vi "main-pressure-logger.vi"() -> ()   [LabVIEW 2016]
uses:
  <vilib>/addons/h5labview2/base/hid_t.ctl
  <vilib>/NI/Modbus Library/API/Wrapper/Create Serial Master.vi
  <vilib>/NI/Modbus Library/API/Master/Modbus Master.lvclass
  <vilib>/NI/Modbus Library/API/Wrapper/API Main.lvlib
  <vilib>/addons/h5labview2/dataset/H5D.lvlib
  <vilib>/addons/h5labview2/file/H5F.lvlib
panel:
  in  "log folder":path=path "C:/Users/LocalAdmin/Documents/omicron-rack/pressure-logs"
  out "Waveform Chart":waveform(sgl)[](graph)
  out "lt":sgl format="%_3e"
  in  "quit":bool
  out "prevacuum":sgl format="%#.3g"
  out "prep":sgl caption="PREP" format="%_3e"
  # "mbar"
  # "mbar"
  # "prep"
  # "lt"
  # "(mbar)"
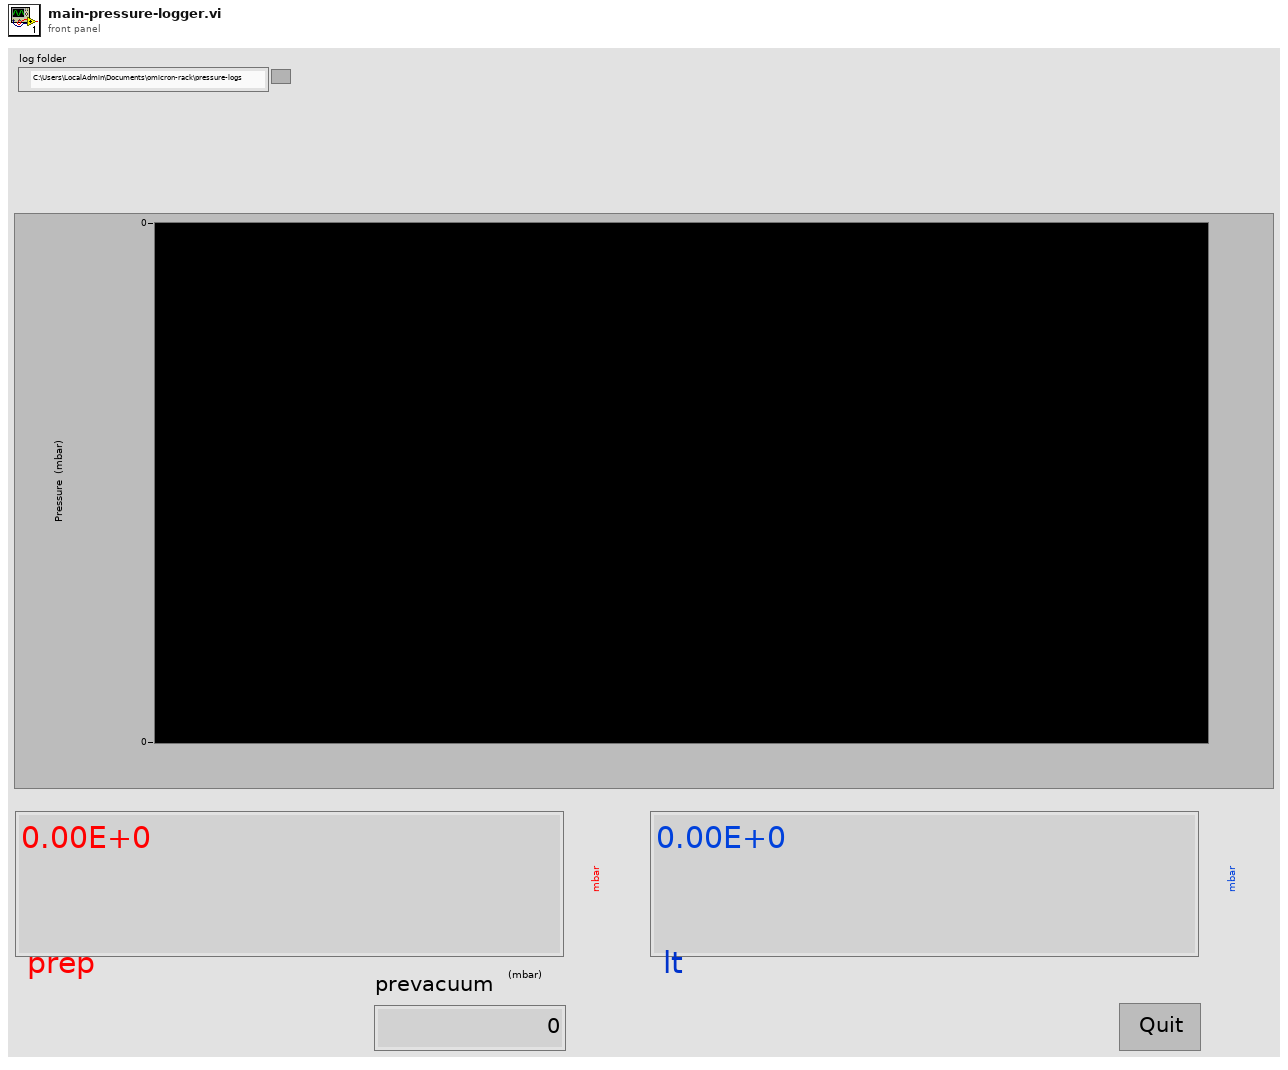
[diagram p1: front panel]
types:
  T1 = typedef "hid_t.ctl" = i32
  T2 = enum16{"open", "replace", "create", "open or create", "replace or create", "replace or create with confirmation"}
  T3 = cluster{"timestamp":i64, "time <19>":string, "prep":sgl, "lt":sgl, "prevacuum":sgl}
  T4 = cluster{"timestamp":i64, "time <19>":string, "prep":sgl, "lt":sgl, "prevacuum":sgl}[]
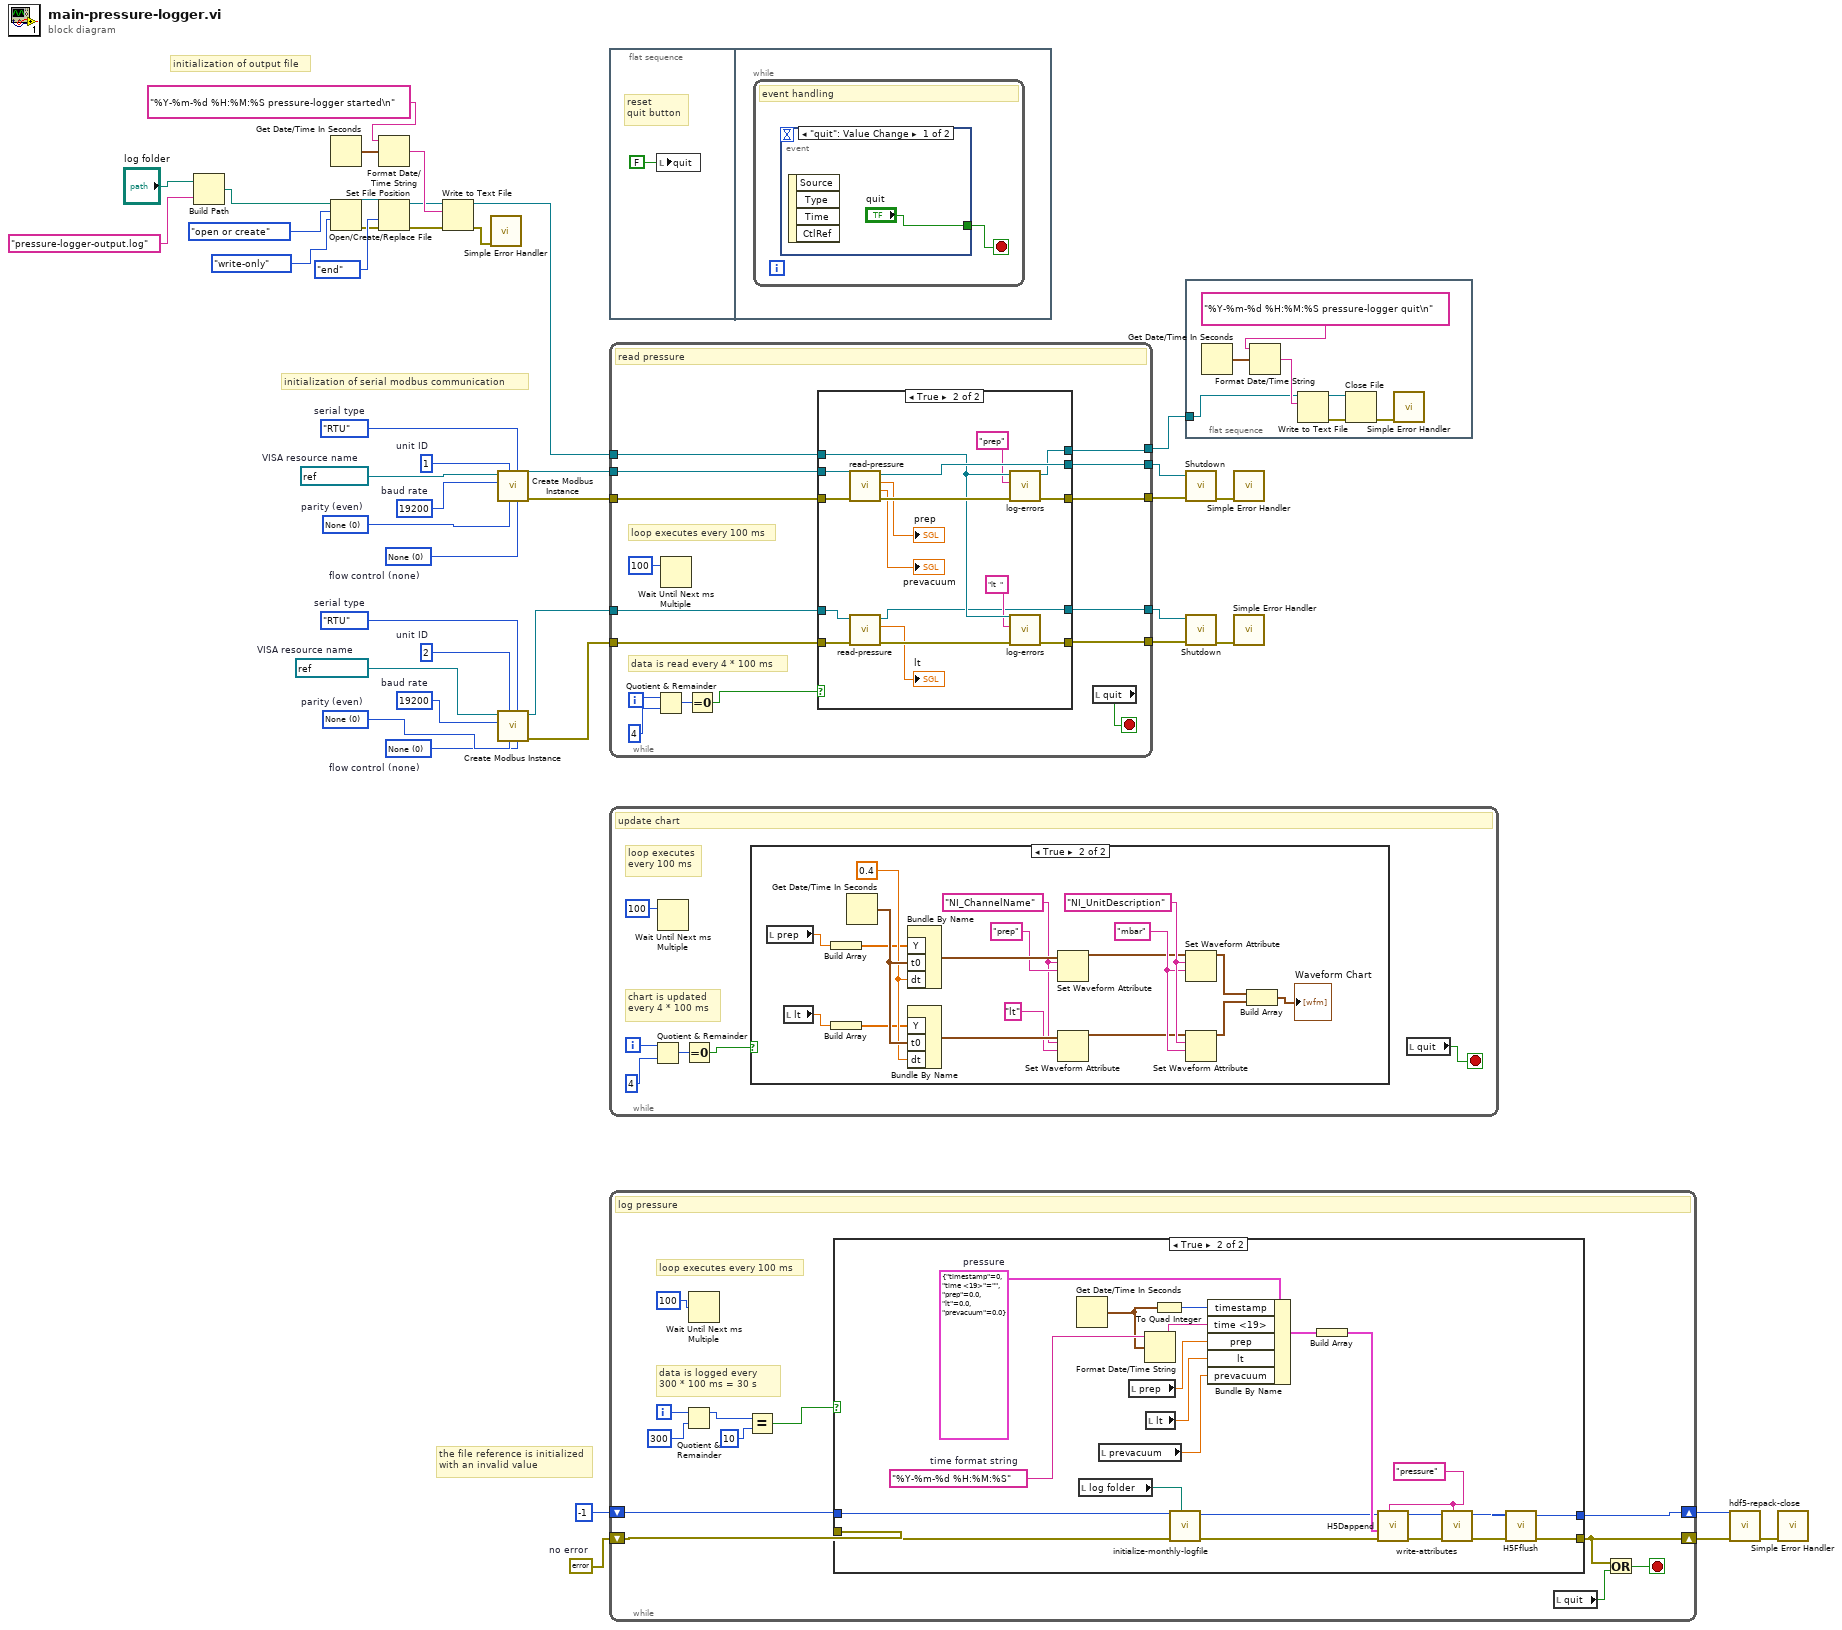
[diagram p0: block diagram]
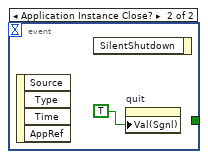
[diagram p3: hidden frame]
diagram:
  w1 = errorcluster {"status"=FALSE, "code"=0, "source"=""}  # no error
  w23 = u16 0 items=["None", "XON/XOFF", "RTS/CTS", "XON/XOFF & RTS/CTS", "DTR/DSR", "XON/XOFF & DTR/DSR"]  # flow control (none)
  w24 = u16 0 items=["None", "Odd", "Even", "Mark", "Space"]  # parity (even)
  w27 = u32 19200  # baud rate
  w28 = refnum<visa-resource-name> "COM12"  # VISA resource name
  w26 = u8 2  # unit ID
  w25 = enum16{"RTU", "ASCII"}."RTU"  # serial type
  w34 = u16 0 items=["None", "XON/XOFF", "RTS/CTS", "XON/XOFF & RTS/CTS", "DTR/DSR", "XON/XOFF & DTR/DSR"]  # flow control (none)
  w35 = u16 0 items=["None", "Odd", "Even", "Mark", "Space"]  # parity (even)
  w38 = u32 19200  # baud rate
  w39 = refnum<visa-resource-name> "COM11"  # VISA resource name
  w37 = u8 1  # unit ID
  w36 = enum16{"RTU", "ASCII"}."RTU"  # serial type
  # "the file reference is initialized\nwith an invalid value"
  # "initialization of serial modbus communication"
  # "initialization of output file"
  n1 = Build Path(base path="log folder", name or relative path="pressure-logger-output.log") -> (appended path=w5:path)
  n2 = Get Date/Time In Seconds() -> (seconds since 1Jan1904=w16:timestamp)
  n3 = Open/Create/Replace File(file path (use dialog)=w5, operation (0:open)=T2."open or create", access (0:read/write)=enum16{"read/write", "read-only", "write-only"}."write-only") -> (refnum out=w32:refnum<file>, error out=w11:errorcluster)  [unwired: 3 in, 1 out]
  n4 = Format Date/Time String(time format string (%c)="%Y-%m-%d %H:%M:%S pressure-logger started\n", seconds (now)=w16) -> (date/time string=w15:string)  [unwired: 1 in]
  n5 = Set File Position(refnum=w32, from (0:start)=enum16{"start", "end", "current"}."end", error in=w11) -> (refnum out=w13:refnum<file>, error out=w10:errorcluster)  [unwired: 1 in]
  n6 = Write to Text File(file (use dialog)=w13, text=w15, error in=w10) -> (refnum out=w12:refnum<file>, error out=w9:errorcluster)  [unwired: 1 in, 1 out]
  n7 = call <vilib>:"Simple Error Handler.vi"("error in (no error)"=w9) -> ()  [unwired: 4 in, 5 out]
  n8 = call-poly <vilib>:"Create Modbus Instance.vi"("flow control (none)"=w34, "serial type"=w36, "parity (even)"=w35, "unit ID"=w37, "baud rate"=w38, "VISA resource name"=w39) -> ("error out"=w42:errorcluster, "serial master instance"=w43:refnum<class "Modbus Master.lvclass">)  [unwired: 4 in]
  n9 = call-poly <vilib>:"Create Modbus Instance.vi"("flow control (none)"=w23, "serial type"=w25, "parity (even)"=w24, "unit ID"=w26, "baud rate"=w27, "VISA resource name"=w28) -> ("error out"=w21:errorcluster, "serial master instance"=w22:refnum<class "Modbus Master.lvclass">)  [unwired: 4 in]
  n10 = flat-sequence {
    frame #0 {
      # "reset\nquit button"
      n11 = local write "quit"(FALSE) -> ()
    }
    frame #1 {
      n12 = while {
        stop <- w45 stop-if-true
        # "event handling"
        n13 = event shown="[0] \"quit\": Value Change" {
          selector: _ -> [_ _]
          dyn-events: _ -> [_ _]
          timeout: _ -> [_ _]
          tunnel: ["quit" _] -> w45
          event "quit": Value Change {
            n14 = event-data() -> ()  [unwired: 1 in, 4 out]
          }
          event Application Instance Close? {
            n15 = event-data() -> ()  [unwired: 1 in, 4 out]
            n16 = event-data() -> ()  [unwired: 2 in, 1 out]
            n17 = property on="quit" class="Bool (strict)"("Val(Sgnl)"=TRUE) -> ()  [unwired: 2 in, 2 out]
          }
        }
      }
    }
  }
  n18 = while {
    tunnel: w22 -> [w51]
    tunnel: w21 -> [w50]
    tunnel: [w49] -> w19
    tunnel: w42 -> [w55]
    tunnel: [w52] -> w40
    tunnel: w43 -> [w56]
    tunnel: [w53] -> w41
    tunnel: w12 -> [w57]
    tunnel: [w54] -> w8
    tunnel: [w48] -> w20
    i -> [w58]
    stop <- w63 stop-if-true
    # "data is read every 4 * 100 ms"
    # "loop executes every 100 ms"
    # "read pressure"
    n19 = Quotient & Remainder(x=w58, y=4) -> (x-y*floor(x/y)=w60:i32)  [unwired: 1 out]
    n20 = Wait Until Next ms Multiple(millisecond multiple=u32 100 ("milliseconds to wait")) -> ()  [unwired: 1 out]
    n21 = Equal To 0?(x=w60) -> (x = 0?=w59:bool)
    n22 = case shown="True" w59 {
      tunnel: w57 -> [w68 w74]
      tunnel: w56 -> [w66 w83]
      tunnel: w55 -> [w67 w82]
      tunnel: [w68 w78] -> w54
      tunnel: [w67 w79] -> w52
      tunnel: [w66 w80] -> w53
      tunnel: w51 -> [w64 w77]
      tunnel: w50 -> [w65 w76]
      tunnel: [w65 w75] -> w49
      tunnel: [w64 w69] -> w48
      frame False {
      }
      frame True {
        n23 = call "read-pressure.vi"("error in"=w82, "Modbus instance in"=w83) -> ("error out"=w85:errorcluster, "Pirani"=→"prevacuum":sgl, "Ion Gauge"=→"prep":sgl, "Modbus instance out"=w80:refnum<class "Modbus Master.lvclass">)  [unwired: 6 in]
        n24 = call "read-pressure.vi"("error in"=w76, "Modbus instance in"=w77) -> ("error out"=w81:errorcluster, "Ion Gauge"=→"lt":sgl, "Modbus instance out"=w69:refnum<class "Modbus Master.lvclass">)  [unwired: 6 in, 1 out]
        n25 = call "log-errors.vi"("error in (no error)"=w85, "device"="prep", "refnum in"=w74) -> ("error out"=w79:errorcluster, "refnum out"=w78:refnum<file>)  [unwired: 7 in]
        n26 = call "log-errors.vi"("error in (no error)"=w81, "device"="lt  ", "refnum in"=w74) -> ("error out"=w75:errorcluster)  [unwired: 7 in, 1 out]
      }
    }
    n27 = local read "quit"() -> (w63:bool)
  }
  n28 = while {
    i -> [w87]
    stop <- w86 stop-if-true
    # "chart is updated\nevery 4 * 100 ms"
    # "loop executes\nevery 100 ms"
    # "update chart"
    n29 = Quotient & Remainder(x=w87, y=4) -> (x-y*floor(x/y)=w89:i32)  [unwired: 1 out]
    n30 = Wait Until Next ms Multiple(millisecond multiple=u32 100 ("milliseconds to wait")) -> ()  [unwired: 1 out]
    n31 = Equal To 0?(x=w89) -> (x = 0?=w88:bool)
    n32 = case shown="True" w88 {
      frame False {
      }
      frame True {
        w96 = "mbar" ("name")
        w97 = "NI_UnitDescription" ("name")
        w103 = "NI_ChannelName" ("name")
        w108 = 0.4 ("dt")
        n33 = local read "prep"() -> (w101:sgl)
        n34 = local read "lt"() -> (w99:sgl)
        n35 = Build Array(w101) -> (w100:sgl[])
        n36 = Build Array(w99) -> (w98:sgl[])
        n37 = Get Date/Time In Seconds() -> (seconds since 1Jan1904=w109:timestamp)
        n38 = Bundle By Name("Y"=w100, "t0"=w109, "dt"=w108) -> (w106:waveform(sgl))  [unwired: 1 in]
        n39 = Bundle By Name("Y"=w98, "t0"=w109, "dt"=w108) -> (w104:waveform(sgl))  [unwired: 1 in]
        n40 = Set Waveform Attribute(5:"prep" ("name"), 6:w103, 7:w106) -> (3:w95:waveform(sgl))  [unwired: 1 in, 2 out]
        n41 = Set Waveform Attribute(5:"lt" ("name"), 6:w103, 7:w104) -> (3:w94:waveform(sgl))  [unwired: 1 in, 2 out]
        n42 = Set Waveform Attribute(5:w96, 6:w97, 7:w95) -> (3:w93:waveform(sgl))  [unwired: 1 in, 2 out]
        n43 = Set Waveform Attribute(5:w96, 6:w97, 7:w94) -> (3:w92:waveform(sgl))  [unwired: 1 in, 2 out]
        n44 = Build Array(w93, w92) -> (→"Waveform Chart":waveform(sgl)[])
      }
    }
    n45 = local read "quit"() -> (w86:bool)
  }
  n46 = while {
    shift-right: [w114] -> w4
    shift-left: T1 -1 ("ref out") -> [w116]
    shift-right: [w113] -> w3
    shift-left: w1 -> [w115]
    i -> [w118]
    stop <- w110 stop-if-true
    # "data is logged every\n300 * 100 ms = 30 s"
    # "loop executes every 100 ms"
    # "log pressure"
    n47 = Quotient & Remainder(x=w118, y=300) -> (x-y*floor(x/y)=w112:i32)  [unwired: 1 out]
    n48 = Wait Until Next ms Multiple(millisecond multiple=u32 100 ("milliseconds to wait")) -> ()  [unwired: 1 out]
    n49 = Equal?(x=w112, y=10) -> (x = y?=w117:bool)
    n50 = case shown="True" w117 {
      tunnel: w116 -> [w123 w131]
      tunnel: w115 -> [w122 w133]
      tunnel: [w123 w141] -> w114
      tunnel: [w122 w142] -> w113
      frame False {
      }
      frame True {
        w140 = "%Y-%m-%d %H:%M:%S"  # time format string
        w125 = "pressure" ("name")
        w145 = T3 {"timestamp"=0, "time <19>"="", "prep"=0.0, "lt"=0.0, "prevacuum"=0.0}  # pressure
        n51 = Get Date/Time In Seconds() -> (seconds since 1Jan1904=w139:timestamp)
        n52 = local read "log folder"() -> (w129:path)
        n53 = local read "prevacuum"() -> (w135:sgl)
        n54 = local read "prep"() -> (w137:sgl)
        n55 = Format Date/Time String(time format string (%c)=w140, seconds (now)=w139) -> (date/time string=w138:string)  [unwired: 1 in]
        n56 = local read "lt"() -> (w136:sgl)
        n57 = To Quad Integer(1:w139) -> (0:w134:i64)
        n58 = call "initialize-monthly-logfile.vi"("log folder"=w129, "error in"=w133, "ref in"=w131) -> ("error out"=w132:errorcluster, "ref out"=w130:T1)  [unwired: 7 in]
        n59 = Bundle By Name(cluster=w145, "timestamp"=w134, "time <19>"=w138, "prep"=w137, "lt"=w136, "prevacuum"=w135) -> (w144:T3)
        n60 = Build Array(w144) -> (w143:T4)
        n61 = call <vilib>:"H5Dappend.vi"("dataset name"=w125, "error in (no error)"=w132, "data"=w143, "ref in"=w130) -> ("error out"=w126:errorcluster, "ref out"=w124:T1)  [unwired: 4 in, 2 out]
        n62 = call "write-attributes.vi"("name"=w125, "error in (no error)"=w126, "ref in"=w124) -> ("error out"=w127:errorcluster, "ref out"=w128:T1)  [unwired: 7 in]
        n63 = call <vilib>:"H5Fflush.vi"("error in (no error)"=w127, "ref in"=w128) -> ("error out"=w142:errorcluster, "ref out"=w141:T1)  [unwired: 8 in]
      }
    }
    n64 = local read "quit"() -> (w121:bool)
    n65 = Or(x=w113, y=w121) -> (x .or. y?=w110:bool)
  }
  n66 = flat-sequence {
    tunnel: w8 -> [w149]
    frame #0 {
      n67 = Get Date/Time In Seconds() -> (seconds since 1Jan1904=w152:timestamp)
      n68 = Format Date/Time String(time format string (%c)="%Y-%m-%d %H:%M:%S pressure-logger quit\n", seconds (now)=w152) -> (date/time string=w151:string)  [unwired: 1 in]
      n69 = Write to Text File(file (use dialog)=w149, text=w151) -> (refnum out=w148:refnum<file>, error out=w147:errorcluster)  [unwired: 2 in, 1 out]
      n70 = Close File(refnum=w148, error in=w147) -> (error out=w146:errorcluster)  [unwired: 1 out]
      n71 = call <vilib>:"Simple Error Handler.vi"("error in (no error)"=w146) -> ()  [unwired: 4 in, 5 out]
    }
  }
  n72 = call-dynamic "Shutdown.vi"("error in"=w40, "Modbus master in"=w41) -> ("error out"=w29:errorcluster)  [unwired: 9 in]
  n73 = call-dynamic "Shutdown.vi"("error in"=w19, "Modbus master in"=w20) -> ("error out"=w18:errorcluster)  [unwired: 9 in]
  n74 = call <vilib>:"Simple Error Handler.vi"("error in (no error)"=w29) -> ()  [unwired: 4 in, 5 out]
  n75 = call <vilib>:"Simple Error Handler.vi"("error in (no error)"=w18) -> ()  [unwired: 4 in, 5 out]
  n76 = call "hdf5-repack-close.vi"("error in"=w3, "ref in"=w4) -> ("error out"=w30:errorcluster)  [unwired: 9 in]
  n77 = call <vilib>:"Simple Error Handler.vi"("error in (no error)"=w30) -> ()  [unwired: 4 in, 5 out]
